vi "TEST(Ganaral Mode).vi"(8 "Error In":errorcluster, 10 "Modbus ID":string, 11 "VISA resource name":refnum<visa-resource-name>) -> (0 "Error Out":errorcluster, 3 "VISA resource name out":refnum<visa-resource-name>)   [LabVIEW 2013]
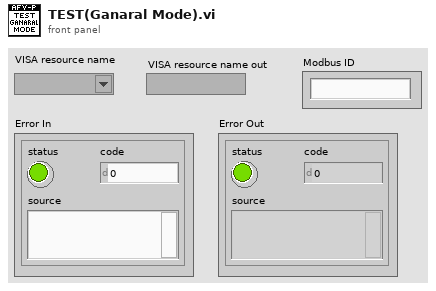
[diagram p1: front panel]
types:
  T1 = cluster{"Length (High)":string, "Length (Low)":string, "Start Address (High)":string, "Start Address (Middle High)":string, "Start Address (Middle Low)":string, "Start Address (Low)":string}
  T2 = cluster{"ID":string, "Function Code":string, "Length (High)":string, "Length (Low)":string, "Start Address (High)":string, "Start Address (Middle High)":string, "Start Address (Middle Low)":string, "Start Address (Low)":string, "Data":string}
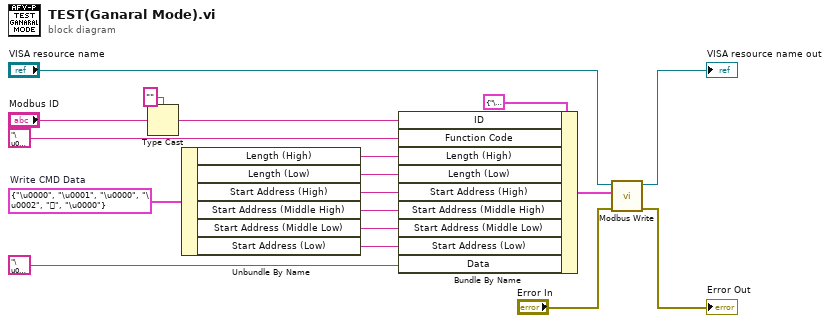
[diagram p0: block diagram]
diagram:
  w11 = T1 {"Length (High)"="\u0000", "Length (Low)"="\u0001", "Start Address (High)"="\u0000", "Start Address (Middle High)"="\u0002", "Start Address (Middle Low)"="", "Start Address (Low)"="\u0000"}  # Write CMD Data
  n1 = Type Cast(type="" ("Binary Data (Hex) 3"), x="Modbus ID") -> (*(type *) &x=w6:string)
  n2 = Unbundle By Name(w11) -> ("Length (High)"=w17:string, "Length (Low)"=w16:string, "Start Address (High)"=w15:string, "Start Address (Middle High)"=w14:string, "Start Address (Middle Low)"=w13:string, "Start Address (Low)"=w12:string)
  n3 = Bundle By Name(cluster=T2 {"ID"="\u0000", "Function Code"="\u0000", "Length (High)"="\u0000", "Length (Low)"="\u0000", "Start Address (High)"="\u0000", "Start Address (Middle High)"="\u0000", "Start Address (Middle Low)"="\u0000", "Start Address (Low)"="\u0000", "Data"=""} ("Write Buffer"), "ID"=w6, "Function Code"="\u0010" ("*(type *) &x"), "Length (High)"=w17, "Length (Low)"=w16, "Start Address (High)"=w15, "Start Address (Middle High)"=w14, "Start Address (Middle Low)"=w13, "Start Address (Low)"=w12, "Data"="\u0006" ("*(type *) &x")) -> (w5:T2)
  n4 = call "Modbus Write.vi"("Error In"="Error In", "Write Buffer"=w5, "VISA resource name"="VISA resource name") -> ("Error Out"=→"Error Out":errorcluster, "VISA resource name out"=→"VISA resource name out":refnum<visa-resource-name>)  [unwired: 7 in]
